vi "AWG_5421_Load_Wfm_Script.vi"(5 "AWG 5421 Inputs":T1={"Resource Name"="AWG_5421", "Sample Rate"=10000000.0, "Trigger Type"=2, "Trigger Source"="PFI0", "Waveform Gain"=0.31, "Digital Filter ON"=TRUE} {"Sample Rate" format="%.2p"; "Trigger Type" items=["None", "Software Edge", "Digital Edge", "Digital Level"]}, 8 "error  in":errorcluster caption="error in", 9 "EXCIT Inputs":T4={"Number of Excitations"=1, "Script Text"="", "Table of Waveforms"=[]} {"Number of Excitations" min=1 max=10}, 10 "SOFTWARE Inputs":T3={"Application Directory"=path "D:/S.O.F.T.S/LABVIEW/PIL", "Software Version"="1.0.0", "Data Path"=path "D:/PIRENEA/DATA", "XML Path"=path "D:/PIRENEA/DATA", "XML File Filter"="*.xml", "XML Saved Path"=path "D:/PIRENEA/DATA/SAVED", "Excit Scripts Path"=path "D:/PIRENEA/TECHNICAL/EXCIT_SCRIPTS", "Excit Scripts File Filter"="*.txt", "Excit Waveforms Path"=path "D:/PIRENEA/TECHNICAL/EXCIT_WFMS", "Excit Waveforms File Filter"="*.bin", "Timing Scripts Path"=path "D:/PIRENEA/TECHNICAL/TIMING_SCRIPTS", "Timing Scripts File Filter"="*.txt", "Timing Waveforms Path"=path "D:/PIRENEA/TECHNICAL/TIMING_WFMS", "Timing Waveforms File Filter"="*.bin", "Trapping Waveforms Path"=path "D:/PIRENEA/TECHNICAL/TRAPPING_WFMS", "Trapping Waveforms File Filter"="*.bin"}, 11 "instrument handle in":refnum<k15>) -> (0 "error out":errorcluster, 1 "Number of Wfms":i32, 2 "FIFO used":i64, 3 "instrument handle out":refnum<k15>, 6 "Script text":string)   [LabVIEW 2024]
doc: "This VI loads the dynamic waveforms and the script into the AWG 5421 board.\n\n1. The waveform binary files are read one by one from the waveform folder.\n2. The data are converted to U32 format and loaded into the on-board memory.\n\nThis VI returns the max memory size of the board, the memory used after loading, and a list of the waveforms loaded. No check of memory overflow is done."
uses:
  controls/EXCIT_Inputs.ctl
  controls/SOFTWARE_Inputs.ctl
  controls/AWG_5421_Inputs.ctl
  <instrlib>/niFgen/niFgen.llb/niFgen_ctl Trigger Source Values (Ring).ctl
  <instrlib>/niFgen/niFgen.llb/niFgen Write Named Waveform (DBL).vi
panel:
  out "FIFO max size":i32
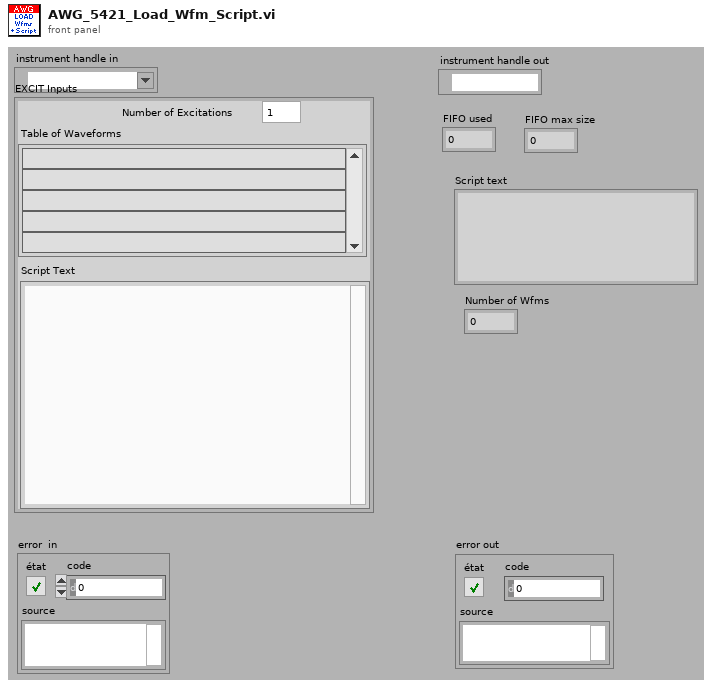
[diagram p1: front panel]
types:
  T1 = typedef "AWG_5421_Inputs.ctl" = cluster{"Resource Name":refnum<k15>, "Sample Rate":dbl, "Trigger Type":u16, "Trigger Source":T2, "Waveform Gain":dbl, "Digital Filter ON":bool}
  T2 = typedef "niFgen_ctl Trigger Source Values (Ring).ctl" = string
  T3 = typedef "SOFTWARE_Inputs.ctl" = cluster{"Application Directory":path, "Software Version":string, "Data Path":path, "XML Path":path, "XML File Filter":string, "XML Saved Path":path, "Excit Scripts Path":path, "Excit Scripts File Filter":string, "Excit Waveforms Path":path, "Excit Waveforms File Filter":string, "Timing Scripts Path":path, "Timing Scripts File Filter":string, "Timing Waveforms Path":path, "Timing Waveforms File Filter":string, "Trapping Waveforms Path":path, "Trapping Waveforms File Filter":string}
  T4 = typedef "EXCIT_Inputs.ctl" = cluster{"Number of Excitations":i32, "Script Text":string, "Table of Waveforms":string[]}
  T5 = enum16{"big-endian, network order", "native, host order", "little-endian"}
  T6 = enum16{"open", "replace", "create", "open or create", "replace or create", "replace or create with confirmation"}
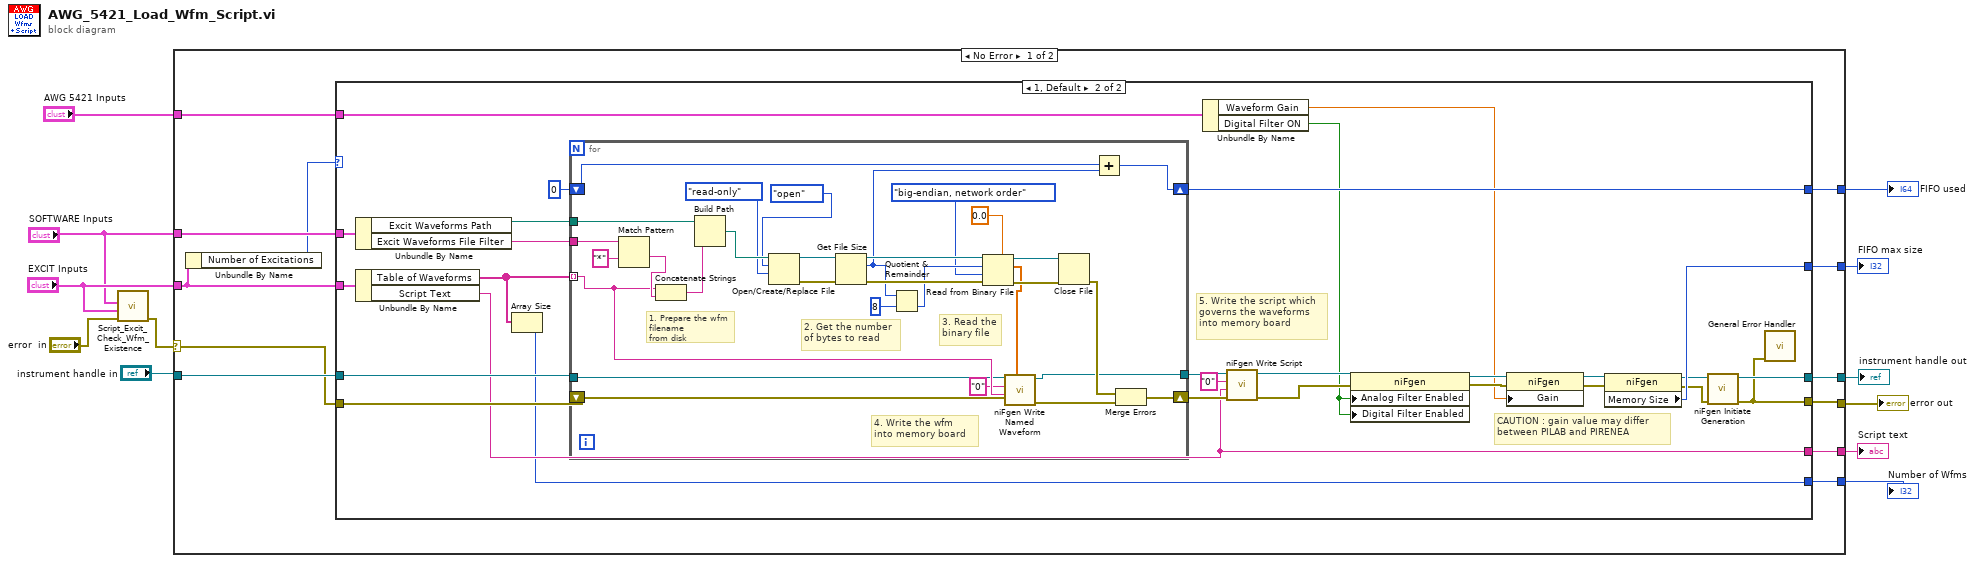
[diagram p0: block diagram]
diagram:
  n1 = call "Script_Excit_Check_Wfm_Existence.vi"("error  in"="error  in", "EXCIT Inputs"="EXCIT Inputs", "SOFTWARE Inputs"="SOFTWARE Inputs") -> ("error out"=w2:errorcluster)  [unwired: 8 in]
  n2 = case shown="No Error" w2 {
    selector: w2 -> [w23 w85]
    tunnel: [w17 w85] -> w12
    tunnel: [w20 w84] -> w8
    tunnel: "instrument handle in" -> [w24 w84]
    tunnel: "SOFTWARE Inputs" -> [w15 _]
    tunnel: "EXCIT Inputs" -> [w13 _]
    tunnel: [w22 _] -> w11
    tunnel: [w21 _] -> w10
    tunnel: [w19 _] -> w7
    tunnel: [w18 _] -> w6
    tunnel: "AWG 5421 Inputs" -> [w16 _]
    frame No Error {
      n3 = Unbundle By Name(w13) -> ("Number of Excitations"=w14:i32)
      n4 = case shown="1, Default" w14 {
        tunnel: w24 -> [_ w53]
        tunnel: w23 -> [w25 w52]
        tunnel: w15 -> [_ w50]
        tunnel: w13 -> [_ w47]
        tunnel: [_ w46] -> w22
        tunnel: [_ w45] -> w21
        tunnel: [_ w39] -> w20
        tunnel: [_ w38] -> w19
        tunnel: [_ w36] -> w18
        tunnel: [w25 w29] -> w17
        tunnel: w16 -> [_ w28]
        frame 0 {
        }
        frame 1, Default {
          # "CAUTION : gain value may differ\nbetween PILAB and PIRENEA"
          # "5. Write the script which\ngoverns the waveforms\ninto memory board"
          n5 = Unbundle By Name(w50) -> ("Excit Waveforms Path"=w49:path, "Excit Waveforms File Filter"=w48:string)
          n6 = Unbundle By Name(w47) -> ("Table of Waveforms"=w37:string[], "Script Text"=w38:string)
          n7 = Array Size(array=w37) -> (size(s)=w36:i32)
          n8 = for {
            shift-right: [w67] -> w44
            shift-left: w52 -> [w61]
            tunnel: w53 -> [w58]
            shift-right: [w70] -> w46
            shift-left: i64 0 -> [w69]
            tunnel: w37 -> [w59] mode=indexing
            tunnel: w49 -> [w66]
            tunnel: w48 -> [w65]
            tunnel: [w57] -> w43
            # "4. Write the wfm\ninto memory board"
            # "3. Read the\nbinary file"
            # "2. Get the number\nof bytes to read"
            # "1. Prepare the wfm filename\nfrom disk"
            n9 = Match Pattern(string=w65, regular expression="*" ("expression régulière")) -> (after substring=w63:string)  [unwired: 1 in, 3 out]
            n10 = Concatenate Strings(w59, w63) -> (w62:string)
            n11 = Build Path(base path=w66, name or relative path=w62) -> (appended path=w81:path)
            n12 = Open/Create/Replace File(file path (use dialog)=w81, operation (0:open)=T6."open", access (0:read/write)=enum16{"read/write", "read-only", "write-only"}."read-only") -> (refnum out=w83:refnum<file>, error out=w82:errorcluster)  [unwired: 3 in, 1 out]
            n13 = Get File Size(file=w83, error in=w82) -> (refnum out=w77:refnum<file>, size (in bytes)=w55:i64, 0:w75:errorcluster)
            n14 = Quotient & Remainder(x=w55, y=i64 8 ("type size (bytes)")) -> (floor(x/y)=w73:i64)  [unwired: 1 out]
            n15 = Read from Binary File(5:0.0 ("data type"), 8:w75, 9:T5."big-endian, network order" ("ordre des octets (0 : big-Endian, network order)"), 10:w73, 11:w77) -> (0:w74:errorcluster, 2:w54:dbl[], 3:w76:refnum<file>)  [unwired: 1 in, 1 out]
            n16 = call-poly <instrlib>:"niFgen Write Named Waveform.vi"("Waveform Data"=w54, "error in (no error)"=w61, "Waveform Name"=w59, "Channel Name"="0", "Instrument Handle"=w58) -> ("error out"=w60:errorcluster, "Instrument Handle Out"=w57:refnum<k15>)  [unwired: 4 in, 1 out]
            n17 = Close File(refnum=w76, error in=w74) -> (error out=w68:errorcluster)  [unwired: 1 out]
            n18 = Add(x=w69, y=w55) -> (x+y=w70:i64)
            n19 = Merge Errors(w68, w60) -> (w67:errorcluster)
          }
          n20 = Unbundle By Name(w28) -> ("Waveform Gain"=w27:dbl, "Digital Filter ON"=w26:bool)
          n21 = call <instrlib>:"niFgen Write Script.vi"("error in (no error)"=w44, "Script"=w38, "Channel Name"="0", "Instrument Handle"=w43) -> ("error out"=w35:errorcluster, "Instrument Handle Out"=w34:refnum<k15>)  [unwired: 6 in]
          n22 = property class="niFgen"(reference=w34, error in=w35, "Analog Filter Enabled"=w26, "Digital Filter Enabled"=w26) -> (reference out=w31:refnum<k15>, error out=w30:errorcluster)
          n23 = property class="niFgen"(reference=w31, error in=w30, "Gain"=w27) -> (reference out=w33:refnum<k15>, error out=w32:errorcluster)
          n24 = property class="niFgen"(reference=w33, error in=w32) -> (reference out=w41:refnum<k15>, error out=w40:errorcluster, "Memory Size"=w45:i32)
          n25 = call <instrlib>:"niFgen Initiate Generation.vi"("error in (no error)"=w40, "Instrument Handle"=w41) -> ("error out"=w29:errorcluster, "Instrument Handle Out"=w39:refnum<k15>)  [unwired: 8 in]
          n26 = call <vilib>:"General Error Handler.vi"("error in (no error)"=w29) -> ()  [unwired: 10 in, 5 out]
        }
      }
    }
    frame Error {
    }
  }
  "error out" <- w12
  "FIFO used" <- w11
  "FIFO max size" <- w10
  "instrument handle out" <- w8
  "Script text" <- w7
  "Number of Wfms" <- w6
